vi "PCE-InfoParser.vi"(7 "Data String":string) -> (8 "Data Cluster":T1 {"Rotateur" format="%.2f"; "Dome" format="%.2f"; "Focus" format="%.2f"; "Année" format="%.2f"; "Temps Universel" format="%<%H:%M:%S%0u>t"; "Temps Sidéral" format="%<%H:%M:%S%0u>t"; "Masse d'air" format="%.2f"; "Epoque" format="%.2f"; "DEC" format="%<%H:%M:%S%0u>t"; "RA" format="%<%H:%M:%S%0u>t"; "HA" format="%<%H:%M:%S%0u>t"})   [LabVIEW 2011]
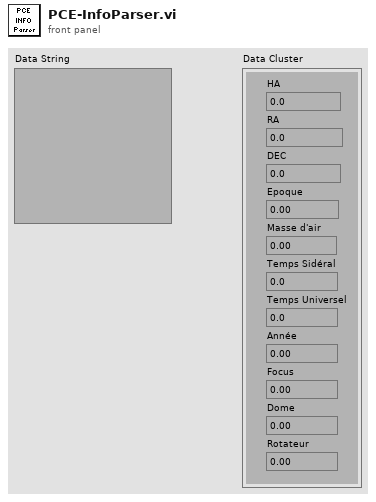
[diagram p1: front panel]
types:
  T1 = cluster{"HA":dbl, "RA":dbl, "DEC":dbl, "Epoque":dbl, "Masse d'air":dbl, "Temps Sidéral":dbl, "Temps Universel":dbl, "Année":dbl, "Focus":dbl, "Dome":dbl, "Rotateur":dbl}
  T2 = cluster{dbl, dbl, dbl, dbl, dbl, dbl, dbl, dbl, dbl, dbl, dbl}
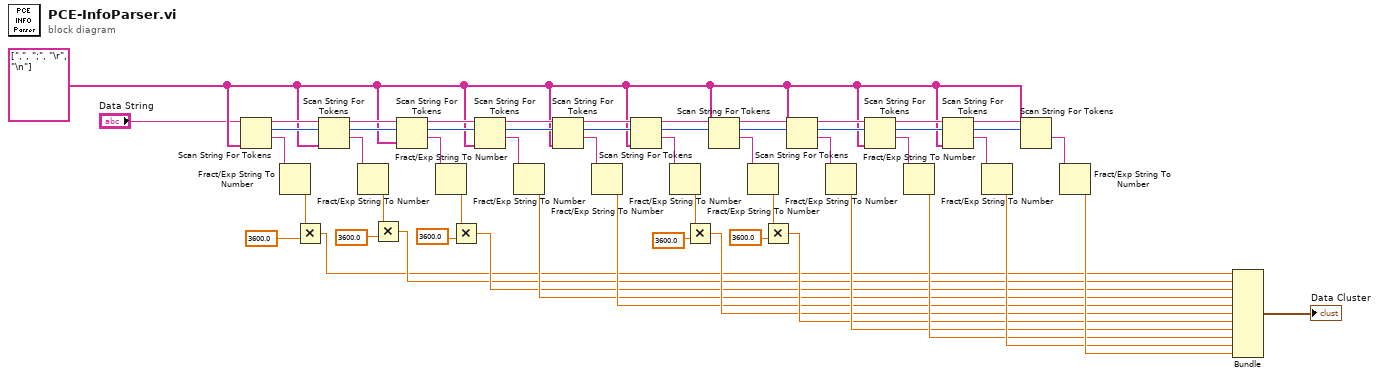
[diagram p0: block diagram]
diagram:
  w14 = string[] [",", ";", "\r", "\n"] ("delimiters (\\s,\\t,\\r,\\n)")
  n1 = Scan String For Tokens(6:w14, 9:"Data String") -> (1:w47:string, 2:w48:i32, 3:w49:string)  [unwired: 4 in, 1 out]
  n2 = Fract/Exp String To Number(string=w47) -> (number=w46:dbl)  [unwired: 3 in, 1 out]
  n3 = Multiply(x=w46, y=3600.0) -> (x*y=w2:dbl)
  n4 = Scan String For Tokens(6:w14, 8:w48, 9:w49) -> (1:w15:string, 2:w51:i32, 3:w50:string)  [unwired: 3 in, 1 out]
  n5 = Fract/Exp String To Number(string=w15) -> (number=w40:dbl)  [unwired: 3 in, 1 out]
  n6 = Multiply(x=w40, y=3600.0) -> (x*y=w3:dbl)
  n7 = Scan String For Tokens(6:w14, 8:w51, 9:w50) -> (1:w43:string, 2:w53:i32, 3:w52:string)  [unwired: 3 in, 1 out]
  n8 = Fract/Exp String To Number(string=w43) -> (number=w38:dbl)  [unwired: 3 in, 1 out]
  n9 = Multiply(x=w38, y=3600.0) -> (x*y=w4:dbl)
  n10 = Scan String For Tokens(6:w14, 8:w53, 9:w52) -> (1:w42:string, 2:w55:i32, 3:w54:string)  [unwired: 3 in, 1 out]
  n11 = Fract/Exp String To Number(string=w42) -> (number=w5:dbl)  [unwired: 3 in, 1 out]
  n12 = Scan String For Tokens(6:w14, 8:w55, 9:w54) -> (1:w41:string, 2:w17:i32, 3:w28:string)  [unwired: 3 in, 1 out]
  n13 = Fract/Exp String To Number(string=w41) -> (number=w6:dbl)  [unwired: 3 in, 1 out]
  n14 = Scan String For Tokens(6:w14, 8:w17, 9:w28) -> (1:w33:string, 2:w31:i32, 3:w32:string)  [unwired: 3 in, 1 out]
  n15 = Fract/Exp String To Number(string=w33) -> (number=w36:dbl)  [unwired: 3 in, 1 out]
  n16 = Multiply(x=w36, y=3600.0) -> (x*y=w7:dbl)
  n17 = Scan String For Tokens(6:w14, 8:w31, 9:w32) -> (1:w34:string, 2:w29:i32, 3:w30:string)  [unwired: 3 in, 1 out]
  n18 = Fract/Exp String To Number(string=w34) -> (number=w37:dbl)  [unwired: 3 in, 1 out]
  n19 = Multiply(x=w37, y=3600.0) -> (x*y=w8:dbl)
  n20 = Scan String For Tokens(6:w14, 8:w29, 9:w30) -> (1:w35:string, 2:w16:i32, 3:w18:string)  [unwired: 3 in, 1 out]
  n21 = Fract/Exp String To Number(string=w35) -> (number=w9:dbl)  [unwired: 3 in, 1 out]
  n22 = Scan String For Tokens(6:w14, 8:w16, 9:w18) -> (1:w21:string, 2:w23:i32, 3:w22:string)  [unwired: 3 in, 1 out]
  n23 = Fract/Exp String To Number(string=w21) -> (number=w10:dbl)  [unwired: 3 in, 1 out]
  n24 = Scan String For Tokens(6:w14, 8:w23, 9:w22) -> (1:w20:string, 2:w25:i32, 3:w24:string)  [unwired: 3 in, 1 out]
  n25 = Fract/Exp String To Number(string=w20) -> (number=w11:dbl)  [unwired: 3 in, 1 out]
  n26 = Scan String For Tokens(6:w14, 8:w25, 9:w24) -> (1:w19:string)  [unwired: 3 in, 3 out]
  n27 = Fract/Exp String To Number(string=w19) -> (number=w12:dbl)  [unwired: 3 in, 1 out]
  n28 = Bundle(w2, w3, w4, w5, w6, w7, w8, w9, w10, w11, w12) -> (→"Data Cluster":T2)  [unwired: 1 in]
